vi "DoorAccess.vi"() -> ()   [LabVIEW 2011]
uses:
  <vilib>/Platform/TimedLoop/XDataNode/timing_clust.ctl
  <vilib>/Platform/TimedLoop/XDataNode/nitl_modes.ctl
  <vilib>/Platform/TimedLoop/XDataNode/wakeup.ctl
  Routine/Queue/Alert.vi
  Routine/Queue/Card.vi
  Variable/gSEL.vi
  Variable/gSIM.vi
  Variable/gSTOP.vi
  <vilib>/Platform/TimedLoop/XDataNode/XDataNode.xnode
  <vilib>/Platform/TimedLoop/XDataNode/XDNodeRunTimeDep.lvlib
  Routine/DoorTread/Tread_02.vi
  Routine/DoorTread/Tread_01.vi
  Routine/DoorTread/Tread_03.vi
  Routine/DoorTread/Alerts.vi
panel:
  out "Certificate":bool
  out "Card Info":string="001001/30305:25197"
  in  "Tab Control":enum32{"Main", "Set 1"}(tab)
  in  "Building":string="A01"
  in  "En0":bool
  out "STA0":bool
  in  "ID 0":u8
  in  "IP 0":string
  in  "Port 0":u16=6341
  in  "En3 3":bool
  out "STA3 3":bool
  in  "ID 5":u8=5
  in  "IP 5":string
  in  "Port 5":u16=1621
  in  "Node 5":u8
  in  "En3 2":bool
  out "STA3 2":bool
  in  "ID 4":u8=4
  in  "IP 4":string
  in  "Port 4":u16=1621
  in  "Node 4":u8
  in  "En3":bool
  in  "En2":bool=TRUE
  in  "En1":bool
  out "STA3":bool
  in  "ID 3":u8=3
  in  "IP 3":string
  in  "Port 3":u16=1621
  in  "Node 3":u8=3
  in  "ID 1":u8=1
  in  "IP 1":string
  in  "Port 1":u16=1621
  in  "Node 1":u8=3
  in  "Node 2":u8=1
  in  "Port 2":u16=1621
  in  "IP 2":string
  in  "ID 2":u8=1
  out "STA2":bool
  out "STA1":bool
  # "Door Access V1.0"
  # "Copyright@2011-2012 Ching-Fu Shipbuilding. All rights reserved."
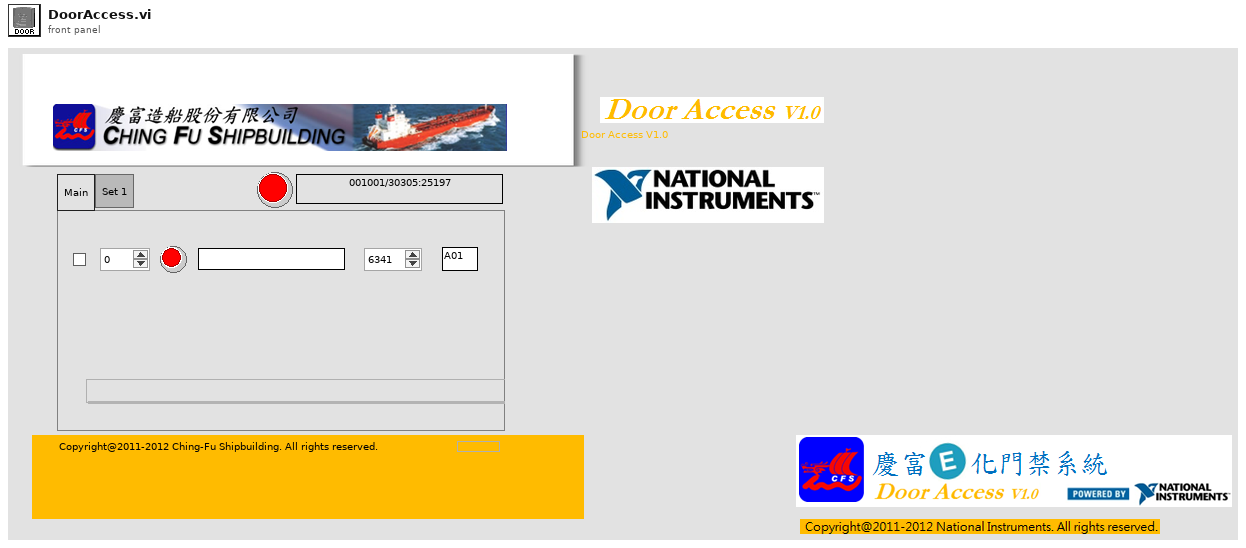
[diagram p1: front panel]
types:
  T1 = enum16{"Obtain", "Enqueue", "Dequeue", "Release"}
  T2 = typedef "XDNodeRunTimeDep.lvlib/timing_clust.ctl" = cluster{"Expected End [f-1]":u64, "Actual End [f-1]":u64, "Finished Late? [f-1]":bool, "Expected End [i-1]":u64, "Actual End [i-1]":u64, "Finished Late? [i-1]":bool, "Expected Start [i]":u64, "Actual Start [i]":u64, "Expected Start [f]":u64, "Actual Start [f]":u64, "Source Name":string, "Structure Name":string, "Period":i64, "Deadline":i64, "Offset":i64, "Start":i64, "Priority":i32, "Timeout":i32, "Mode":T3, "Wakeup Reason":T4, "Error":errorcluster, "Source Type":string, "Secondary Source Type":string, "Global End Time":u64, "Global Start Time":u64, "Frame Duration":u64, "Iteration Duration":u64, "Assigned CPU":i32, "I/O Scan Engine Mode":u32}
  T3 = typedef "XDNodeRunTimeDep.lvlib/nitl_modes.ctl" = enum32{"No Change", "Process missed periods, maintain original phase", "Discard missed periods, maintain original phase", "Process missed periods, ignore original phase", "Discard missed periods, ignore original phase"}
  T4 = typedef "XDNodeRunTimeDep.lvlib/wakeup.ctl" = enum32{"Normal", "Aborted", "Asynchronous wakeup", "Timing source error", "Timed loop error", "Timeout"}
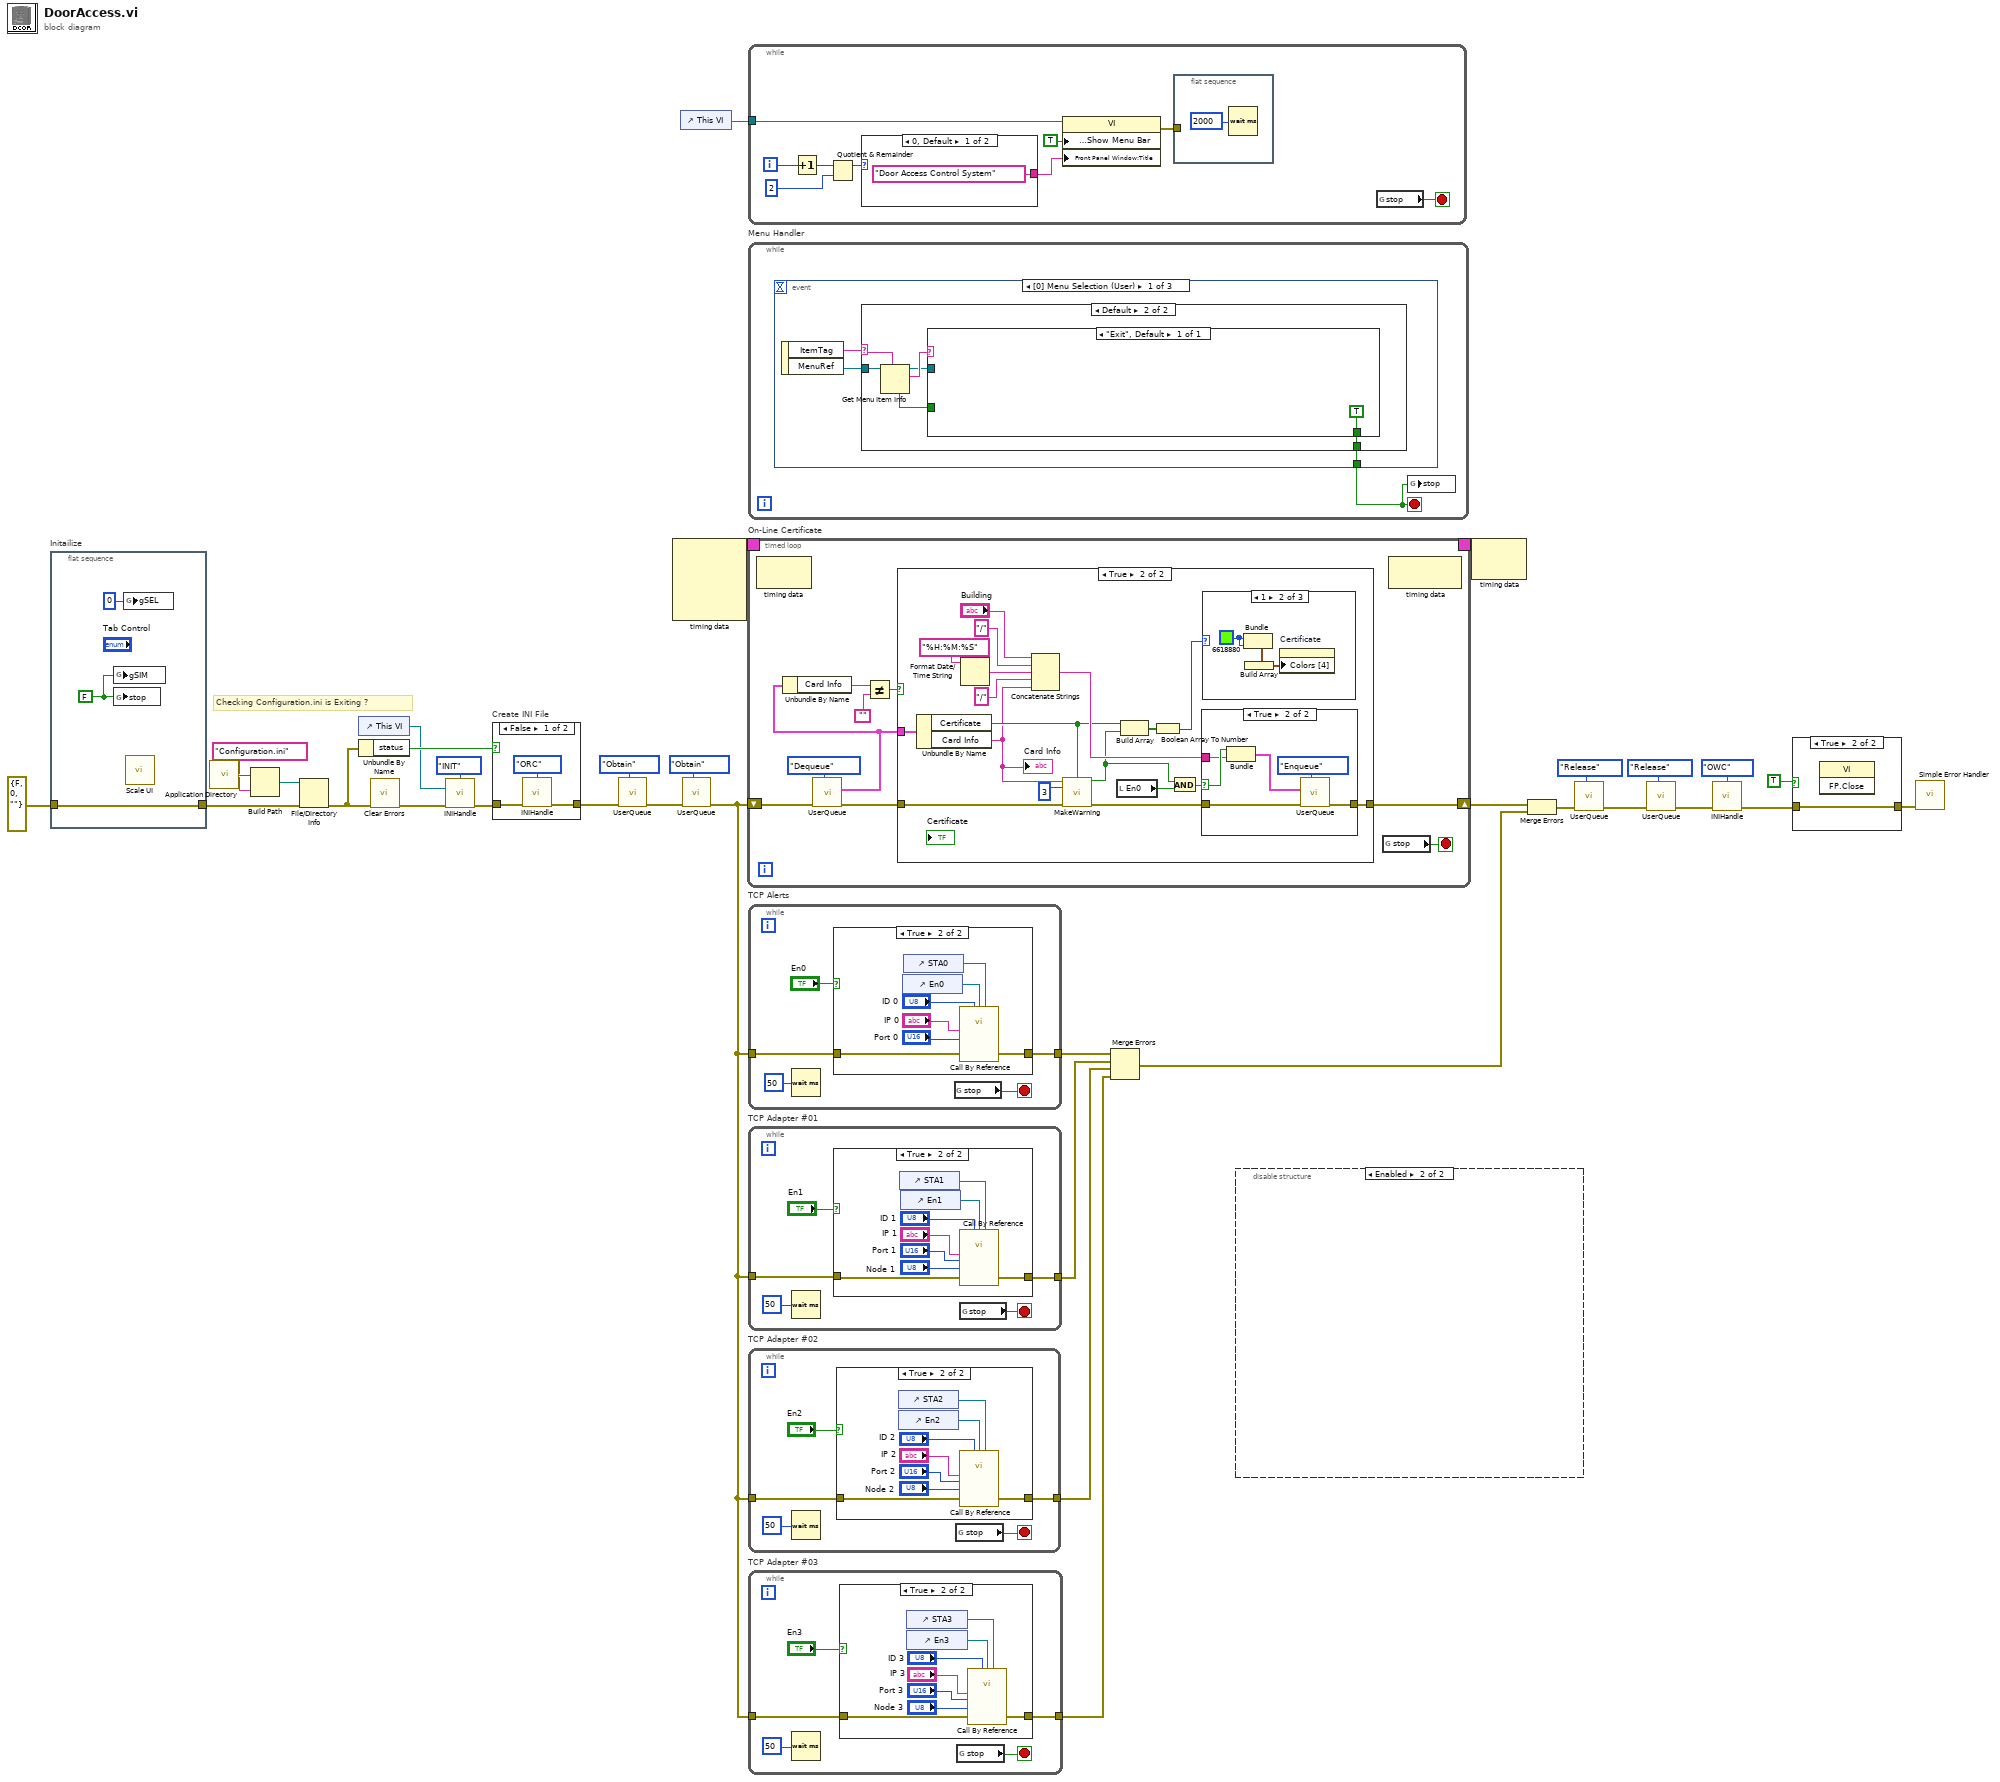
[diagram p0: block diagram]
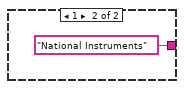
[diagram p3: hidden frame]
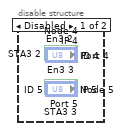
[diagram p4: hidden frame]
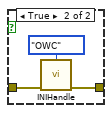
[diagram p5: hidden frame]
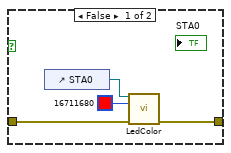
[diagram p6: hidden frame]
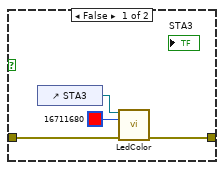
[diagram p7: hidden frame]
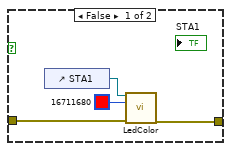
[diagram p8: hidden frame]
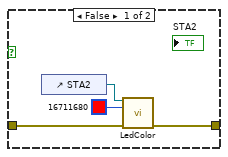
[diagram p9: hidden frame]
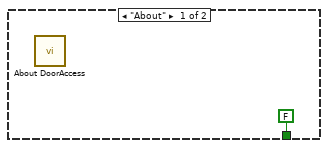
[diagram p10: hidden frame]
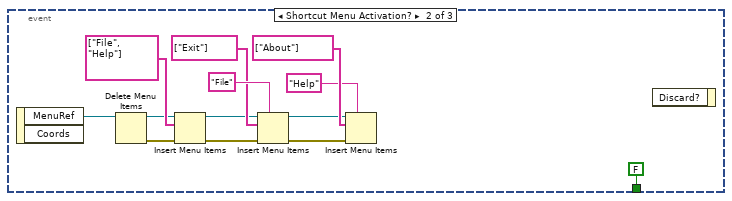
[diagram p11: hidden frame]
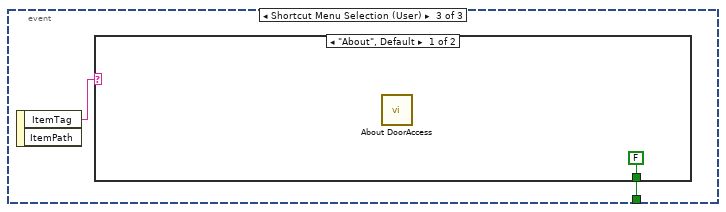
[diagram p12: hidden frame]
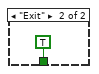
[diagram p13: hidden frame]
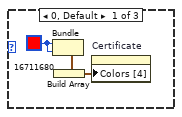
[diagram p15: hidden frame]
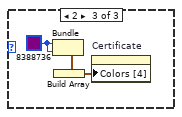
[diagram p16: hidden frame]
diagram:
  # "Checking Configuration.ini is Exiting ?"
  n1 = flat-sequence "Initailize" {
    tunnel: errorcluster {"status"=FALSE, "code"=0, "source"=""} ("error constant") -> [w35]
    tunnel: [w35] -> w23
    frame #0 {
      w36 = FALSE ("stop")
      n2 = global write "gSIM.vi" "gSIM"(w36) -> ()
      n3 = global write "gSTOP.vi" "stop"(w36) -> ()
      n4 = global write "gSEL.vi" "gSEL"(0 ("gSEL")) -> ()
      n5 = call "Scale UI.vi"() -> ()  [unwired: 12 in]
    }
  }
  n6 = call <vilib>:"Application Directory.vi"() -> ("Application Directory"=w15:path)
  n7 = Build Path(base path=w15, name or relative path="Configuration.ini") -> (appended path=w16:path)
  n8 = File/Directory Info(path=w16, error in=w23) -> (error out=w12:errorcluster)  [unwired: 6 out]
  n9 = control-ref of="This VI"() -> (w8:refnum<vi>)
  n10 = Unbundle By Name(w12) -> ("status"=w13:bool)
  n11 = call <vilib>:"Clear Errors.vi"("error in (no error)"=w12) -> ("error out"=w10:errorcluster)  [unwired: 6 in]
  n12 = call "INIHandle.vi"("Mode"=enum16{"INIT", "OWC", "ORC"}."INIT", "VI Refnum"=w8, "error in (no error)"=w10) -> ("error out"=w9:errorcluster)  [unwired: 12 in]
  n13 = case "Create INI File" shown="False" w13 {
    tunnel: w9 -> [w39 w42]
    tunnel: [w38 w41] -> w2
    frame False {
      n14 = call "INIHandle.vi"("Mode"=enum16{"INIT", "OWC", "ORC"}."ORC", "error in (no error)"=w39) -> ("error out"=w38:errorcluster)  [unwired: 13 in]
    }
    frame True {
      n15 = call "INIHandle.vi"("Mode"=enum16{"INIT", "OWC", "ORC"}."OWC", "error in (no error)"=w42) -> ("error out"=w41:errorcluster)  [unwired: 13 in]
    }
  }
  n16 = call-poly "UserQueue.vi"("Mode"=T1."Obtain", "error in (no error)"=w2) -> ("error out"=w27:errorcluster)  [unwired: 8 in, 1 out]
  n17 = node-c288() -> (w30:T2)  [unwired: 4 in]
  n18 = control-ref of="This VI"() -> (w6:refnum<vi>)
  n19 = call-poly "UserQueue.vi"("Mode"=T1."Obtain", "error in (no error)"=w27) -> ("error out"=w22:errorcluster)  [unwired: 8 in, 1 out]
  n20 = timed-loop "On-Line Certificate" {
    shift-right: [w47] -> w31
    shift-left: w22 -> [w51]
    timing: w30 -> [_]
    timing-out: [_] -> w29
    stop <- w44 stop-if-true
    n21 = node-c288() -> ()  [unwired: 1 in, 1 out]
    n22 = call-poly "UserQueue.vi"("Mode"=T1."Dequeue", "error in (no error)"=w51) -> ("error out"=w48:errorcluster, "Queue Out"=w46:cluster{"Certificate":bool, "Card Info":string})  [unwired: 8 in]
    n23 = Unbundle By Name(w46) -> ("Card Info"=w50:string)
    n24 = Not Equal?(x=w50, y="") -> (x != y?=w49:bool)
    n25 = case shown="True" w49 {
      tunnel: w48 -> [w55 w61]
      tunnel: [w55 w72] -> w47
      tunnel: w46 -> [_ w73]
      frame False {
      }
      frame True {
        n26 = Unbundle By Name(w73) -> ("Certificate"=w57:bool, "Card Info"=w56:string)
        "Card Info" <- w56
        n27 = Format Date/Time String(time format string (%c)="%H:%M:%S") -> (date/time string=w63:string)  [unwired: 2 in]
        n28 = Concatenate Strings("Building", "/", w63, "/", w56) -> (w66:string)
        n29 = call "MakeWarning.vi"("String"=w56, "Enable"=w57, "Setup"=u8 3, "error in"=w61) -> ("Warning"=w58:bool, "error out"=w60:errorcluster)  [unwired: 10 in]
        n30 = local read "En0"() -> (w68:bool)
        n31 = Build Array(w57, w58) -> (w70:bool[])
        n32 = Boolean Array To Number(Boolean array=w70) -> (number=w69:u32)
        n33 = And(x=w58, y=w68) -> (x .and. y?=w71:bool)
        n34 = case shown="True" w71 {
          selector: w71 -> [_ w86]
          tunnel: w60 -> [w83 w88]
          tunnel: [w83 w87] -> w72
          tunnel: w66 -> [_ w85]
          frame False {
          }
          frame True {
            n35 = Bundle(w86, w85) -> (w84:cluster{bool, string})  [unwired: 1 in]
            n36 = call-poly "UserQueue.vi"("Mode"=T1."Enqueue", "error in (no error)"=w88, "Queue In"=w84) -> ("error out"=w87:errorcluster)  [unwired: 7 in, 1 out]
          }
        }
        n37 = case shown="1" w69 {
          frame 0, Default {
            w76 = u32 16711680 ("Color Box")
            n38 = Bundle("Color Box"=w76, "Color Box"=w76) -> (w75:cluster{"Color Box":u32, "Color Box":u32})  [unwired: 1 in]
            n39 = Build Array(w75) -> (w74:cluster{"Color Box":u32, "Color Box":u32}[])
            n40 = property on="Certificate" class="Bool (strict)"("Colors [4]"=w74) -> ()  [unwired: 2 in, 2 out]
          }
          frame 1 {
            w79 = u32 6618880 ("Color Box")
            n41 = Bundle("Color Box"=w79, "Color Box"=w79) -> (w78:cluster{"Color Box":u32, "Color Box":u32})  [unwired: 1 in]
            n42 = Build Array(w78) -> (w77:cluster{"Color Box":u32, "Color Box":u32}[])
            n43 = property on="Certificate" class="Bool (strict)"("Colors [4]"=w77) -> ()  [unwired: 2 in, 2 out]
          }
          frame 2 {
            w82 = u32 8388736 ("Color Box")
            n44 = Bundle("Color Box"=w82, "Color Box"=w82) -> (w81:cluster{"Color Box":u32, "Color Box":u32})  [unwired: 1 in]
            n45 = Build Array(w81) -> (w80:cluster{"Color Box":u32, "Color Box":u32}[])
            n46 = property on="Certificate" class="Bool (strict)"("Colors [4]"=w80) -> ()  [unwired: 2 in, 2 out]
          }
        }
      }
    }
    n47 = global read "gSTOP.vi" "stop"() -> (w44:bool)
    n48 = node-c288() -> ()  [unwired: 1 in, 1 out]
  }
  n49 = while {
    tunnel: w6 -> [w97]
    i -> [w91]
    stop <- w98 stop-if-true
    n50 = Increment(x=w91) -> (x+1=w92:i32)
    n51 = Quotient & Remainder(x=w92, y=2) -> (x-y*floor(x/y)=w95:i32)  [unwired: 1 out]
    n52 = case shown="0, Default" w95 {
      tunnel: ["Door Access Control System" "National Instruments"] -> w94
      frame 0, Default {
      }
      frame 1 {
      }
    }
    n53 = property class="VI"(reference=w97, "Front Panel Window:Show Menu Bar"=TRUE, "Front Panel Window:Title"=w94) -> (error out=w90:errorcluster)  [unwired: 1 in, 1 out]
    n54 = flat-sequence {
      tunnel: w90 -> [_]
      frame #0 {
        n55 = Wait (ms)(milliseconds to wait=u32 2000) -> ()  [unwired: 1 out]
      }
    }
    n56 = global read "gSTOP.vi" "stop"() -> (w98:bool)
  }
  n57 = while "Menu Handler" {
    stop <- w102 stop-if-true
    n58 = event shown="[0] Menu Selection (User)" {
      selector: _ -> [_ _ _]
      dyn-events: _ -> [_ _ _]
      timeout: _ -> [_ _ _]
      tunnel: [w103 FALSE w127] -> w102
      event Menu Selection (User) {
        n59 = event-data() -> ("ItemTag"=w104:string, "MenuRef"=w105:refnum<k9>)  [unwired: 1 in]
        n60 = case shown="Default" w104 {
          selector: w104 -> [_ w111]
          tunnel: w105 -> [_ w112]
          tunnel: [FALSE w109] -> w103
          frame "About" {
            n61 = call "About DoorAccess.vi"() -> ()  [unwired: 1 out]
          }
          frame Default {
            n62 = Get Menu Item Info(7:w111, 11:w112) -> (2:w110:string, 3:w108:refnum<k9>, 4:w107:bool)  [unwired: 1 in, 4 out]
            n63 = case shown="\"Exit\", Default" w110 {
              tunnel: [TRUE] -> w109
              tunnel: w108 -> [_]
              tunnel: w107 -> [_]
              frame "Exit", Default {
              }
            }
          }
        }
      }
      event Shortcut Menu Activation? {
        n64 = event-data() -> ("MenuRef"=w115:refnum<k9>)  [unwired: 1 in, 1 out]
        n65 = Delete Menu Items(9:w115) -> (0:w119:errorcluster, 3:w116:refnum<k9>)  [unwired: 3 in]
        n66 = Insert Menu Items(6:w119, 8:string[] ["File", "Help"] ("item names"), 9:w116) -> (0:w120:errorcluster, 3:w118:refnum<k9>)  [unwired: 3 in, 1 out]
        n67 = Insert Menu Items(5:"File" ("menu tag"), 6:w120, 8:string[] ["Exit"] ("item names"), 9:w118) -> (0:w123:errorcluster, 3:w124:refnum<k9>)  [unwired: 2 in, 1 out]
        n68 = Insert Menu Items(5:"Help" ("menu tag"), 6:w123, 8:string[] ["About"] ("item names"), 9:w124) -> ()  [unwired: 2 in, 3 out]
        n69 = event-data() -> ()  [unwired: 2 in, 1 out]
      }
      event Shortcut Menu Selection (User) {
        n70 = event-data() -> ("ItemTag"=w128:string)  [unwired: 1 in, 1 out]
        n71 = case shown="\"About\", Default" w128 {
          tunnel: [FALSE TRUE] -> w127
          frame "About", Default {
            n72 = call "About DoorAccess.vi"() -> ()  [unwired: 1 out]
          }
          frame "Exit" {
          }
        }
      }
    }
    n73 = global write "gSTOP.vi" "stop"(w102) -> ()
  }
  n74 = while "TCP Alerts" {
    tunnel: w22 -> [w134]
    tunnel: [w133] -> w21
    stop <- w132 stop-if-true
    n75 = Wait (ms)(milliseconds to wait=u32 50) -> ()  [unwired: 1 out]
    n76 = case shown="True" "En0" {
      tunnel: w134 -> [w137 w141]
      tunnel: [w138 w140] -> w133
      frame False {
        n77 = control-ref of="STA0"() -> (w136:refnum<vi>)
        n78 = call "LedColor.vi"("Boolean in"=w136, "Color Box"=u32 16711680, "error in (no error)"=w137) -> ("error out"=w138:errorcluster)  [unwired: 12 in]
      }
      frame True {
        n79 = control-ref of="En0"() -> (w146:refnum<vi>)
        n80 = control-ref of="STA0"() -> (w145:refnum<vi>)
        n81 = call-by-ref "?"("IP"="IP 0", "ID"="ID 0", "EnRefnum"=w146, "StRefnum"=w145, "Port"="Port 0", "error in (no error)"=w141) -> ("error out"=w140:errorcluster)  [unwired: 11 in, 2 out]
      }
    }
    n82 = global read "gSTOP.vi" "stop"() -> (w132:bool)
  }
  n83 = while "TCP Adapter #01" {
    tunnel: w22 -> [w150]
    tunnel: [w149] -> w20
    stop <- w148 stop-if-true
    n84 = Wait (ms)(milliseconds to wait=u32 50) -> ()  [unwired: 1 out]
    n85 = case shown="True" "En1" {
      tunnel: w150 -> [w153 w163]
      tunnel: [w154 w159] -> w149
      frame False {
        n86 = control-ref of="STA1"() -> (w152:refnum<vi>)
        n87 = call "LedColor.vi"("Boolean in"=w152, "Color Box"=u32 16711680, "error in (no error)"=w153) -> ("error out"=w154:errorcluster)  [unwired: 12 in]
      }
      frame True {
        n88 = control-ref of="STA1"() -> (w157:refnum<vi>)
        n89 = control-ref of="En1"() -> (w156:refnum<vi>)
        n90 = call-by-ref "?"("IP"="IP 1", "ID"="ID 1", "EnRefnum"=w156, "StRefnum"=w157, "Port"="Port 1", "Number"="Node 1", "error in (no error)"=w163) -> ("error out"=w159:errorcluster)  [unwired: 10 in, 2 out]
      }
    }
    n91 = global read "gSTOP.vi" "stop"() -> (w148:bool)
  }
  n92 = while "TCP Adapter #02" {
    tunnel: w22 -> [w168]
    tunnel: [w167] -> w19
    stop <- w165 stop-if-true
    n93 = Wait (ms)(milliseconds to wait=u32 50) -> ()  [unwired: 1 out]
    n94 = case shown="True" "En2" {
      tunnel: w168 -> [w171 w175]
      tunnel: [w170 w174] -> w167
      frame False {
        n95 = control-ref of="STA2"() -> (w169:refnum<vi>)
        n96 = call "LedColor.vi"("Boolean in"=w169, "Color Box"=u32 16711680, "error in (no error)"=w171) -> ("error out"=w170:errorcluster)  [unwired: 12 in]
      }
      frame True {
        n97 = control-ref of="STA2"() -> (w176:refnum<vi>)
        n98 = control-ref of="En2"() -> (w173:refnum<vi>)
        n99 = call-by-ref "?"("IP"="IP 2", "ID"="ID 2", "EnRefnum"=w173, "StRefnum"=w176, "Port"="Port 2", "Number"="Node 2", "error in (no error)"=w175) -> ("error out"=w174:errorcluster)  [unwired: 10 in, 2 out]
      }
    }
    n100 = global read "gSTOP.vi" "stop"() -> (w165:bool)
  }
  n101 = while "TCP Adapter #03" {
    tunnel: w22 -> [w185]
    tunnel: [w184] -> w18
    stop <- w182 stop-if-true
    n102 = Wait (ms)(milliseconds to wait=u32 50) -> ()  [unwired: 1 out]
    n103 = case shown="True" "En3" {
      tunnel: w185 -> [w189 w197]
      tunnel: [w188 w192] -> w184
      frame False {
        n104 = control-ref of="STA3"() -> (w186:refnum<vi>)
        n105 = call "LedColor.vi"("Boolean in"=w186, "Color Box"=u32 16711680, "error in (no error)"=w189) -> ("error out"=w188:errorcluster)  [unwired: 12 in]
      }
      frame True {
        n106 = control-ref of="STA3"() -> (w191:refnum<vi>)
        n107 = control-ref of="En3"() -> (w190:refnum<vi>)
        n108 = call-by-ref "?"("IP"="IP 3", "ID"="ID 3", "EnRefnum"=w190, "StRefnum"=w191, "Port"="Port 3", "Number"="Node 3", "error in (no error)"=w197) -> ("error out"=w192:errorcluster)  [unwired: 10 in, 2 out]
      }
    }
    n109 = global read "gSTOP.vi" "stop"() -> (w182:bool)
  }
  n110 = Merge Errors(w21, w20, w19, w18) -> (w17:errorcluster)
  n111 = disable-structure shown="Enabled" {
    frame Disabled {
    }
    frame Enabled {
    }
  }
  n112 = node-c288(w29) -> ()  [unwired: 1 out]
  n113 = Merge Errors(w31, w17) -> (w32:errorcluster)
  n114 = call-poly "UserQueue.vi"("Mode"=T1."Release", "error in (no error)"=w32) -> ("error out"=w25:errorcluster)  [unwired: 8 in, 1 out]
  n115 = call-poly "UserQueue.vi"("Mode"=T1."Release", "error in (no error)"=w25) -> ("error out"=w7:errorcluster)  [unwired: 8 in, 1 out]
  n116 = call "INIHandle.vi"("Mode"=enum16{"INIT", "OWC", "ORC"}."OWC", "error in (no error)"=w7) -> ("error out"=w1:errorcluster)  [unwired: 13 in]
  n117 = case shown="True" TRUE {
    tunnel: w1 -> [w198 w199]
    tunnel: [w198 w199] -> w3
    frame False {
    }
    frame True {
      n118 = invoke class="VI" method="FP.Close"() -> ()  [unwired: 3 in, 3 out]
    }
  }
  n119 = call <vilib>:"Simple Error Handler.vi"("error in (no error)"=w3) -> ()  [unwired: 4 in, 5 out]
